vi "SetStatus.vi"(8 "error in (no error)":errorcluster, 10 "Status":T1, 11 "reference in":refnum<class "TestView_Tree_Single.lvclass">) -> (0 "error out":errorcluster, 3 "reference in":refnum<class "TestView_Tree_Single.lvclass">)   [LabVIEW 2022 SP3, in "TestView_Tree_Single.lvlib" / "TestView_Tree_Single.lvclass"]
uses:
  TestView_Tree_Single.lvclass
  Components/TestView_Base.lvlibp/ViewStatus.ctl
  Components/TestView_Base.lvlibp/TestView_Base.lvclass
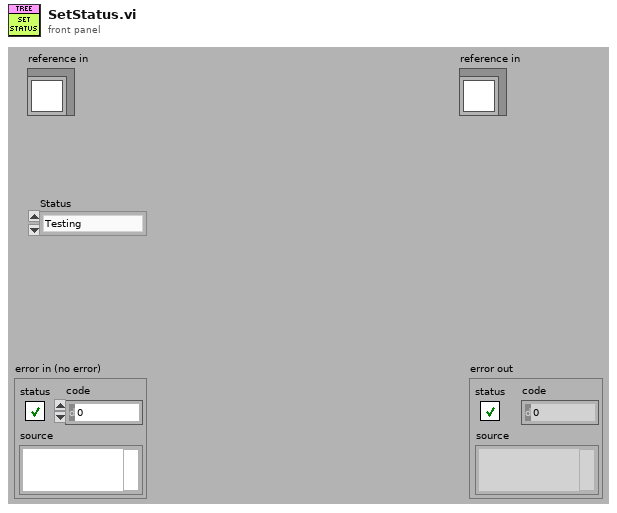
[diagram p1: front panel]
types:
  T1 = typedef "TestView_Base.lvlibp/TestView_Base.lvclass/ViewStatus.ctl" = enum16{"Testing", "Ready", "Logout", "Login", "PASS", "FAIL", "FAULT", "ABORTED"}
  T2 = typedef "TestView_Tree_Single.lvlib/TestView_Tree_Single.lvclass/ObjectAttributes.ctl" = cluster{"Front Panel":refnum<vi>, "Last_Item":string, "Config":T3, "Title":string, "User":string, "TreeRef":refnum<vi>, "Active DUT":i32, "Status":T1, "SN":string, "Spec":string}
  T3 = typedef "TestView_Tree_Single.lvlib/TestView_Tree_Single.lvclass/Config.ctl" = cluster{"default":string}
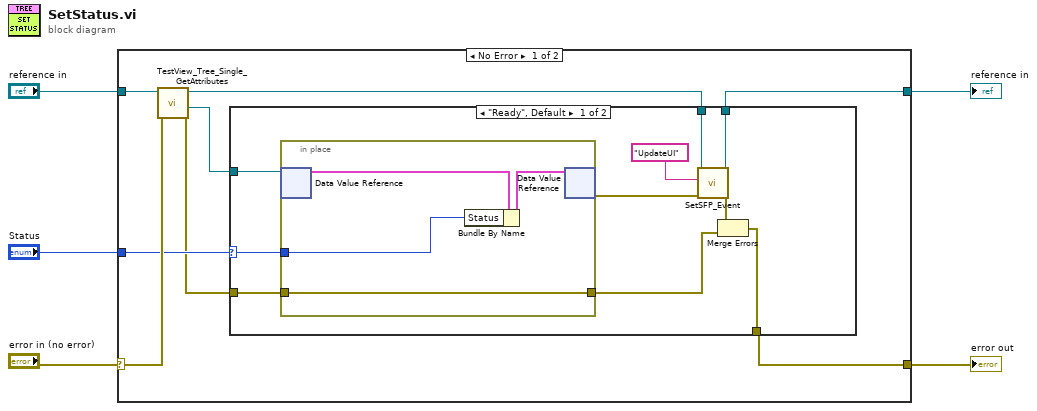
[diagram p0: block diagram]
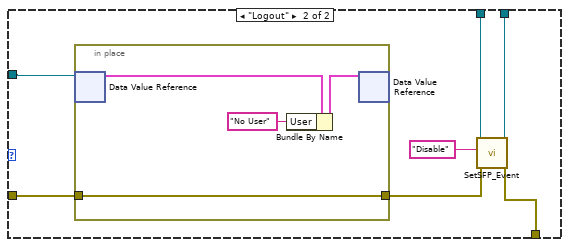
[diagram p2: hidden frame]
diagram:
  n1 = case shown="No Error" "error in (no error)" {
    selector: "error in (no error)" -> [w13 w40]
    tunnel: [w8 w40] -> w2
    tunnel: [w6 w39] -> w4
    tunnel: "reference in" -> [w12 w39]
    tunnel: "Status" -> [w10 _]
    frame No Error {
      n2 = call "TestView_Tree_Single_GetAttributes.vi"("error in (no error)"=w13, "reference in"=w12) -> ("error out"=w9:errorcluster, "DataRef"=w11:refnum<data-value>, "reference out"=w7:refnum<class "TestView_Tree_Single.lvclass">)  [unwired: 6 in, 1 out]
      n3 = case shown="\"Ready\", Default" w10 {
        selector: w10 -> [w16 _]
        tunnel: w11 -> [w23 w30]
        tunnel: [w20 w34] -> w8
        tunnel: w7 -> [w19 w33]
        tunnel: [w18 w32] -> w6
        tunnel: w9 -> [w15 w29]
        frame "Ready", Default {
          n4 = in-place {
            in-place-border: w16 -> [w24]
            in-place-border: [w25] -> w14
            in-place-border: w15 -> [w25]
            n5 = in-place-dvr #1(w23) -> (w26:T2)  [unwired: 1 out]
            n6 = Bundle By Name(cluster=w26, "Status"=w24) -> (w27:T2)
            n7 = in-place-dvr #1(w27) -> (w22:errorcluster)  [unwired: 1 out]
          }
          n8 = call-dynamic "SetSFP_Event.vi"("error in (no error)"=w22, "msg"="UpdateUI", "reference in"=w19) -> ("error out"=w21:errorcluster, "reference out"=w18:refnum<class "TestView_Tree_Single.lvclass">)  [unwired: 7 in]
          n9 = Merge Errors(w21, w14) -> (w20:errorcluster)
        }
        frame "Logout" {
          n10 = in-place {
            in-place-border: [w35] -> w28
            in-place-border: w29 -> [w35]
            n11 = in-place-dvr #2(w30) -> (w37:T2)  [unwired: 1 out]
            n12 = Bundle By Name(cluster=w37, "User"="No User") -> (w38:T2)
            n13 = in-place-dvr #2(w38) -> ()  [unwired: 2 out]
          }
          n14 = call-dynamic "SetSFP_Event.vi"("error in (no error)"=w28, "msg"="Disable", "reference in"=w33) -> ("error out"=w34:errorcluster, "reference out"=w32:refnum<class "TestView_Tree_Single.lvclass">)  [unwired: 7 in]
        }
      }
    }
    frame Error {
    }
  }
  "error out" <- w2
  "reference in" <- w4
